vi "ValidateFilePath.vi"(11 "File Path In":path) -> (1 "Valid File Path?":bool, 3 "File Path Out":path)   [LabVIEW 2016]
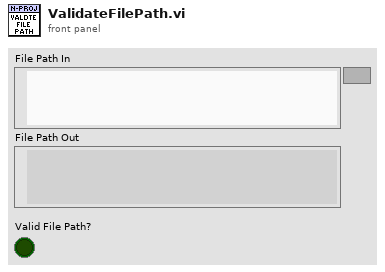
[diagram p1: front panel]
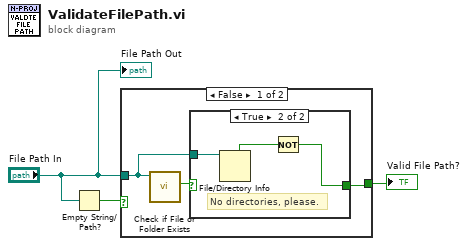
[diagram p0: block diagram]
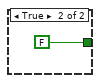
[diagram p3: hidden frame]
diagram:
  n1 = Empty String/Path?(string/path="File Path In") -> (empty?=w3:bool)
  n2 = case shown="False" w3 {
    tunnel: [w5 FALSE ("Valid Path?")] -> w2
    tunnel: "File Path In" -> [w4 _]
    frame False {
      n3 = call <vilib>:"Check if File or Folder Exists.vi"("path"=w4) -> ("file or folder exists?"=w6:bool)  [unwired: 8 in, 2 out]
      n4 = case shown="True" w6 {
        selector: w6 -> [w7 _]
        tunnel: [w7 w8] -> w5
        tunnel: w4 -> [_ w10]
        frame False {
        }
        frame True {
          # "No directories, please."
          n5 = File/Directory Info(path=w10) -> (directory=w9:bool)  [unwired: 1 in, 6 out]
          n6 = Not(x=w9) -> (.not. x?=w8:bool)
        }
      }
    }
    frame True {
    }
  }
  "Valid File Path?" <- w2
  "File Path Out" <- "File Path In"
